vi "Create Task.vi"(8 "error in":errorcluster, 10 "Task name":string="AnalogOutputTask", 11 "NI Analog Output in":refnum<class "NI Analog Output.lvclass">) -> (0 "error out":errorcluster, 3 "NI Analog Output out":refnum<class "NI Analog Output.lvclass">)   [LabVIEW 2023, in "HardwareAbstractionLayer_LVOOP.lvlib" / "NI Analog Output.lvclass"]
doc: "This VI DAQmx Create Auto Task"
uses:
  NI Analog Output.lvclass
  NI Analog Output.lvclass/NI Analog Output.ctl
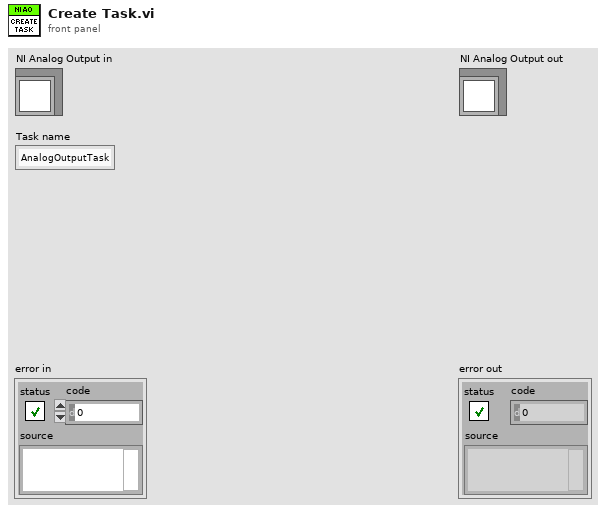
[diagram p1: front panel]
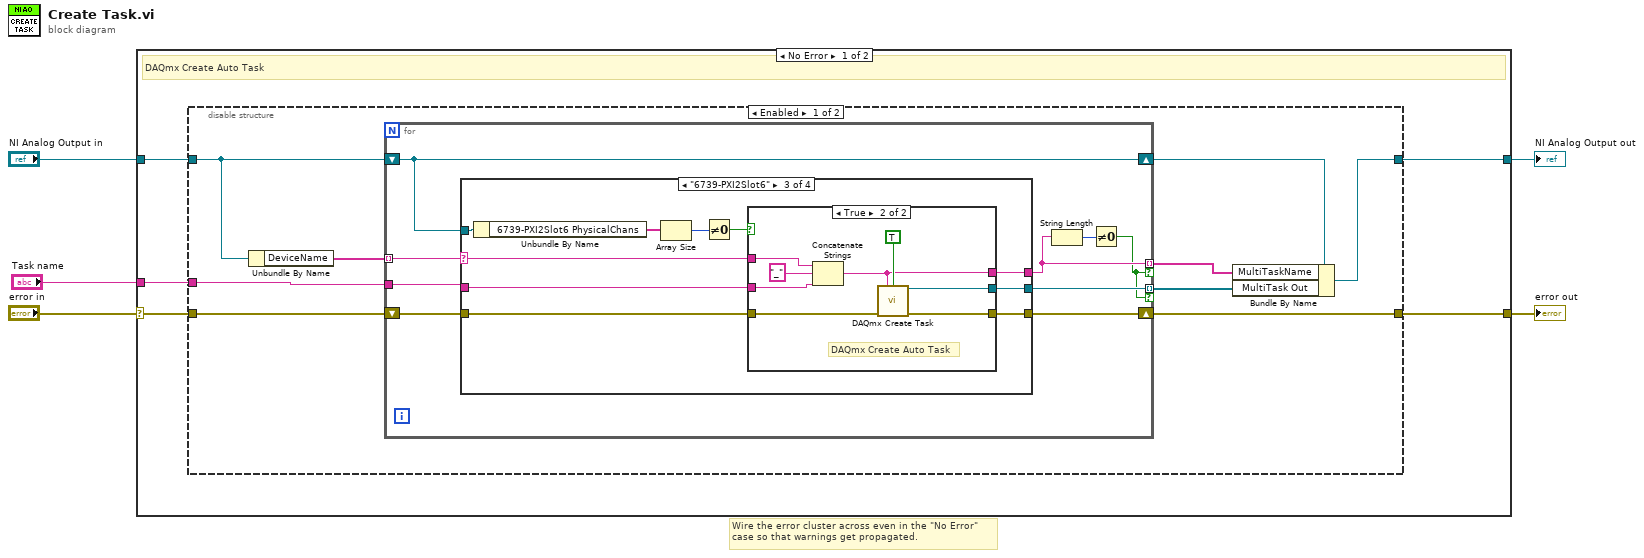
[diagram p0: block diagram]
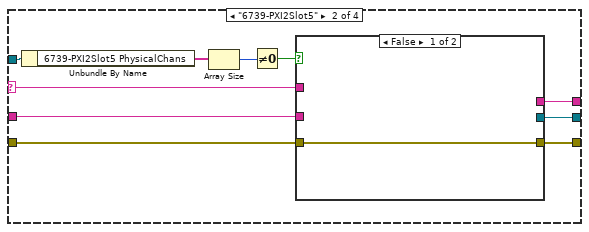
[diagram p3: hidden frame]
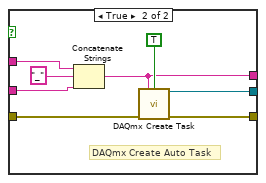
[diagram p4: hidden frame]
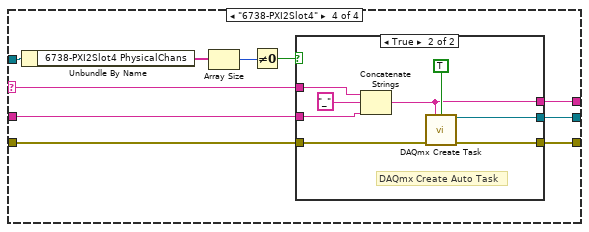
[diagram p6: hidden frame]
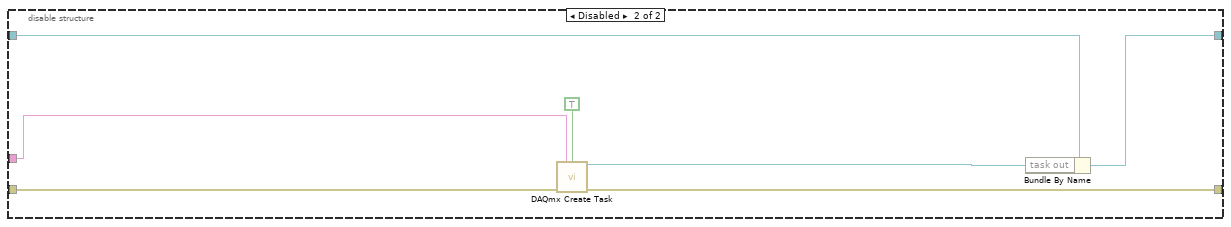
[diagram p8: hidden frame]
diagram:
  # "Wire the error cluster across even in the \"No Error\"\ncase so that warnings get propagated."
  n1 = case shown="No Error" "error in" {
    selector: "error in" -> [w10 w95]
    tunnel: [w9 w95] -> w4
    tunnel: [w8 w94] -> w2
    tunnel: "NI Analog Output in" -> [w6 w94]
    tunnel: "Task name" -> [w7 _]
    frame No Error {
      # "DAQmx Create Auto Task"
      n2 = disable-structure shown="Enabled" {
        disable-tunnel: w10 -> [w19 w92]
        disable-tunnel: [w18 w91] -> w9
        disable-tunnel: [w17 w87] -> w8
        disable-tunnel: w7 -> [w15 w90]
        disable-tunnel: w6 -> [w12 w89]
        frame Enabled {
          n3 = Unbundle By Name(w12) -> ("DeviceName"=w14:tag[])
          n4 = for {
            tunnel: [w26] -> w16 mode=indexing if=w20
            tunnel: w15 -> [w25]
            shift-right: [w27] -> w18
            shift-left: w19 -> [w28]
            tunnel: w14 -> [w24] mode=indexing
            tunnel: [w22] -> w13 mode=indexing if=w20
            shift-right: [w23] -> w11
            shift-left: w12 -> [w23]
            n5 = case shown="\"6739-PXI2Slot6\"" w24 {
              selector: w24 -> [_ w35 w54 w73]
              tunnel: w28 -> [w29 w39 w58 w77]
              tunnel: [w29 w38 w57 w76] -> w27
              tunnel: [_ w37 w56 w75] -> w26
              tunnel: w25 -> [_ w36 w55 w74]
              tunnel: [_ w34 w53 w72] -> w22
              tunnel: w23 -> [_ w33 w52 w71]
              frame "", Default {
              }
              frame "6739-PXI2Slot5" {
                n6 = Unbundle By Name(w33) -> ("6739-PXI2Slot5 PhysicalChans"=w31:tag[])
                n7 = Array Size(array=w31) -> (size(s)=w30:i32)
                n8 = Not Equal To 0?(x=w30) -> (x != 0?=w32:bool)
                n9 = case shown="False" w32 {
                  tunnel: w39 -> [w40 w48]
                  tunnel: [w40 w47] -> w38
                  tunnel: [_ w46] -> w37
                  tunnel: w36 -> [_ w44]
                  tunnel: w35 -> [_ w43]
                  tunnel: [_ w41] -> w34
                  frame False {
                  }
                  frame True {
                    # "DAQmx Create Auto Task"
                    n10 = Concatenate Strings(w43, "_", w44) -> (w41:string)
                    n11 = call <vilib>:"DAQmx Create Task.vi"("new task name"=w41, "auto cleanup"=TRUE, "error in"=w48) -> ("task out"=w46:refnum<k21>, "error out"=w47:errorcluster)  [unwired: 11 in]
                  }
                }
              }
              frame "6739-PXI2Slot6" {
                n12 = Unbundle By Name(w52) -> ("6739-PXI2Slot6 PhysicalChans"=w50:tag[])
                n13 = Array Size(array=w50) -> (size(s)=w49:i32)
                n14 = Not Equal To 0?(x=w49) -> (x != 0?=w51:bool)
                n15 = case shown="True" w51 {
                  tunnel: w58 -> [w59 w67]
                  tunnel: [w59 w66] -> w57
                  tunnel: [_ w65] -> w56
                  tunnel: w55 -> [_ w63]
                  tunnel: w54 -> [_ w62]
                  tunnel: [_ w60] -> w53
                  frame False {
                  }
                  frame True {
                    # "DAQmx Create Auto Task"
                    n16 = Concatenate Strings(w62, "_", w63) -> (w60:string)
                    n17 = call <vilib>:"DAQmx Create Task.vi"("new task name"=w60, "auto cleanup"=TRUE, "error in"=w67) -> ("task out"=w65:refnum<k21>, "error out"=w66:errorcluster)  [unwired: 11 in]
                  }
                }
              }
              frame "6738-PXI2Slot4" {
                n18 = Unbundle By Name(w71) -> ("6738-PXI2Slot4 PhysicalChans"=w69:tag[])
                n19 = Array Size(array=w69) -> (size(s)=w68:i32)
                n20 = Not Equal To 0?(x=w68) -> (x != 0?=w70:bool)
                n21 = case shown="True" w70 {
                  tunnel: w77 -> [w78 w86]
                  tunnel: [w78 w85] -> w76
                  tunnel: [_ w84] -> w75
                  tunnel: w74 -> [_ w82]
                  tunnel: w73 -> [_ w81]
                  tunnel: [_ w79] -> w72
                  frame False {
                  }
                  frame True {
                    # "DAQmx Create Auto Task"
                    n22 = Concatenate Strings(w81, "_", w82) -> (w79:string)
                    n23 = call <vilib>:"DAQmx Create Task.vi"("new task name"=w79, "auto cleanup"=TRUE, "error in"=w86) -> ("task out"=w84:refnum<k21>, "error out"=w85:errorcluster)  [unwired: 11 in]
                  }
                }
              }
            }
            n24 = String Length(string=w22) -> (length=w21:i32)
            n25 = Not Equal To 0?(x=w21) -> (x != 0?=w20:bool)
          }
          n26 = Bundle By Name(cluster=w11, "MultiTaskName"=w13, "MultiTask Out"=w16) -> (w17:refnum<class "NI Analog Output.lvclass">)
        }
        frame Disabled {
          n27 = call <vilib>:"DAQmx Create Task.vi"("new task name"=w90, "auto cleanup"=TRUE, "error in"=w92) -> ("task out"=w88:refnum<k21>, "error out"=w91:errorcluster)  [unwired: 11 in]
          n28 = Bundle By Name(cluster=w89, "task out"=w88) -> (w87:refnum<class "NI Analog Output.lvclass">)
        }
      }
    }
    frame Error {
    }
  }
  "error out" <- w4
  "NI Analog Output out" <- w2
